vi "SLSC Convert EDS Command to VS Channel.vi"(0 "command":T3, 5 "Physical Channel":string) -> (4 "name":string, 6 "Channel":T1, 8 "SLSC Command Name":string, 10 "documentation-en":string, 14 "description-en":string)   [LabVIEW 2015, in "SLSC CD System Explorer.lvlib"]
uses:
  SLSC CD System Explorer.lvlib
  SLSC EDS API/JSON parsing/command.ctl
  <vilib>/NI Veristand/Custom Device API/Custom Device Channel.ctl
  <vilib>/NI Veristand/Custom Device API/Custom Device Channel Type.ctl
  <vilib>/NI VeriStand/Custom Device API/Custom Device API.lvlib
  SLSC CD Shared/SLSC CD Shared.lvlib
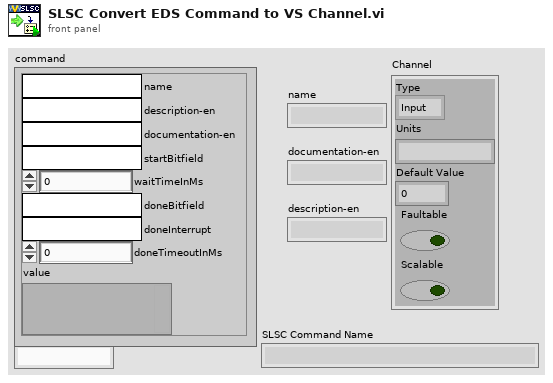
[diagram p1: front panel]
types:
  T1 = typedef "Custom Device API.lvlib/Custom Device Channel.ctl" = cluster{"Type":T2, "Units":string, "Default Value":dbl, "Faultable":bool, "Scalable":bool}
  T2 = typedef "Custom Device API.lvlib/Custom Device Channel Type.ctl" = enum16{"Input", "Output"}
  T3 = typedef "command.ctl" = cluster{"name":string, "description-en":string, "documentation-en":string, "startBitfield":string, "waitTimeInMs":i32, "doneBitfield":string, "doneInterrupt":string, "doneTimeoutInMs":i32, "value":variant}
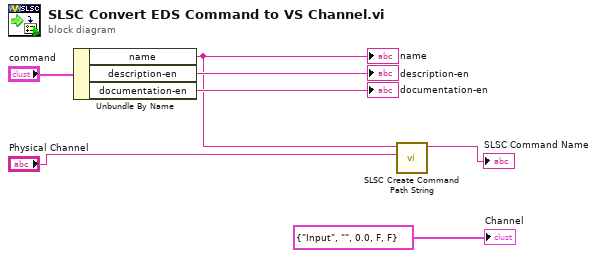
[diagram p0: block diagram]
diagram:
  n1 = Unbundle By Name("command") -> ("name"=w3:string, "description-en"=→"description-en":string, "documentation-en"=→"documentation-en":string)
  "name" <- w3
  n2 = call "SLSC Create Command Path String.vi"("Physical Channel"="Physical Channel", "name"=w3) -> ("SLSC Path String"=→"SLSC Command Name":string)  [unwired: 9 in]
  "Channel" <- T1 {"Type"=enum."Input", "Units"="", "Default Value"=0.0, "Faultable"=FALSE, "Scalable"=FALSE} ("Channel")
